vi "Execute Loaded Command.vi"(8 "error in (no error)":errorcluster, 11 "Command Handler in":refnum<class "Command Handler.lvclass">) -> (0 "error out":errorcluster, 2 "Stop":bool, 3 "Command Handler out":refnum<class "Command Handler.lvclass">)   [LabVIEW 2017, in "Command Handler.lvlib" / "Command Handler.lvclass"]
uses:
  Command Handler.lvclass
  Command Handler.lvclass/Command Handler.ctl
  Command Handler Messages/Command Handler Global API/Command Handler Global.vi
  Command Parents/Command.lvclass
  Command Handler.lvlib
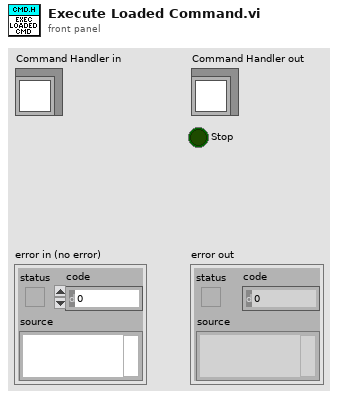
[diagram p1: front panel]
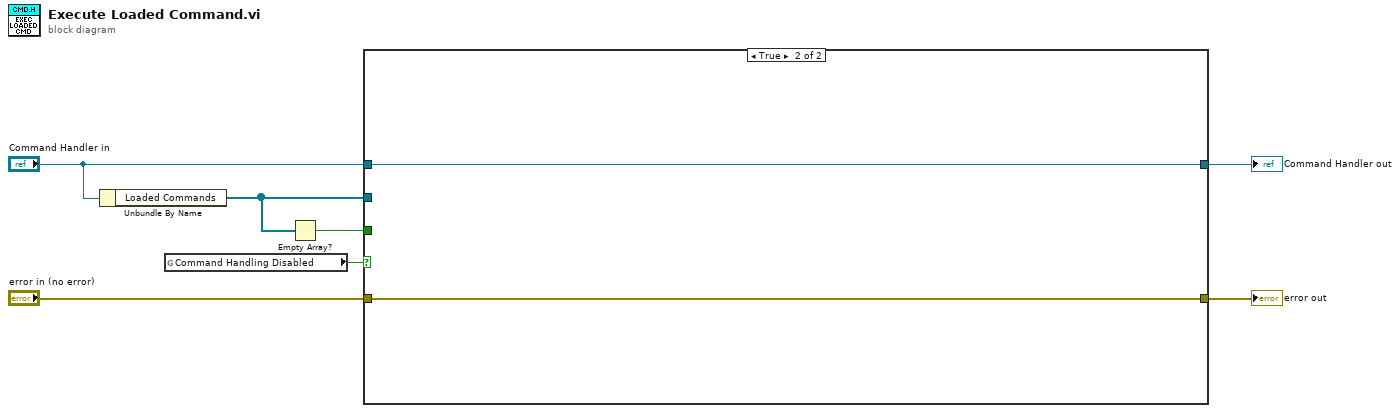
[diagram p0: block diagram]
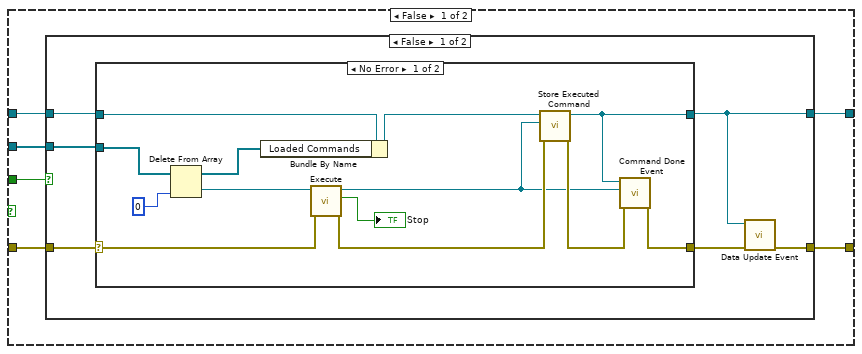
[diagram p2: hidden frame]
diagram:
  n1 = Unbundle By Name("Command Handler in") -> ("Loaded Commands"=w3:refnum<class "Command.lvclass">[])
  n2 = global read "Command Handler Global.vi" "Command Handling Disabled"() -> (w1:bool)
  n3 = Empty Array?(array=w3) -> (empty?=w2:bool)
  n4 = case shown="True" w1 {
    tunnel: "error in (no error)" -> [w13 w37]
    tunnel: [w12 w38] -> w6
    tunnel: [w11 w37] -> w5
    tunnel: "Command Handler in" -> [w10 w38]
    tunnel: w3 -> [w9 _]
    tunnel: w2 -> [w8 _]
    frame False {
      n5 = case shown="False" w8 {
        tunnel: w13 -> [w19 w35]
        tunnel: [w15 w36] -> w12
        tunnel: [w16 w35] -> w11
        tunnel: w10 -> [w18 w36]
        tunnel: w9 -> [w17 _]
        frame False {
          n6 = case shown="No Error" w19 {
            selector: w19 -> [w32 w34]
            tunnel: [w22 w34] -> w14
            tunnel: [w21 w33] -> w15
            tunnel: w18 -> [w29 w33]
            tunnel: w17 -> [w26 _]
            frame No Error {
              n7 = Delete From Array(array=w26, index=0) -> (deleted portion=w27:refnum<class "Command.lvclass">, array with subset deleted=w24:refnum<class "Command.lvclass">[])  [unwired: 1 in]
              n8 = Bundle By Name(cluster=w29, "Loaded Commands"=w24) -> (w25:refnum<class "Command Handler.lvclass">)
              n9 = call-dynamic "Execute.vi"("error in (no error)"=w32, "Command in"=w27) -> ("error out"=w31:errorcluster, "Stop"=→"Stop":bool, "Command out"=w20:refnum<class "Command.lvclass">)  [unwired: 7 in]
              n10 = call-dynamic "Store Executed Command.vi"("error in (no error)"=w31, "Completed Command"=w20, "Command Handler in"=w25) -> ("error out"=w23:errorcluster, "Command Handler out"=w21:refnum<class "Command Handler.lvclass">)  [unwired: 7 in]
              n11 = call "Command Done Event.vi"("error in (no error)"=w23, "Command In"=w20, "Command Handler in"=w21) -> ("error out"=w22:errorcluster)  [unwired: 8 in]
            }
            frame Error {
            }
          }
          n12 = call "Data Update Event.vi"("error in (no error)"=w14, "Command Handler in"=w15) -> ("error out"=w16:errorcluster)  [unwired: 9 in]
        }
        frame True {
        }
      }
    }
    frame True {
    }
  }
  "error out" <- w5
  "Command Handler out" <- w6
